vi "UI 3 Error.vi"(8 "error in (no error)":errorcluster, 11 "Data":variant) -> (0 "error out":errorcluster)   [LabVIEW 2018, in "Error Handler.lvlib"]
doc: "This subVI enqueues the named action in to the communications queue along with the input data."
uses:
  Error Handler.lvlib
  Private Controls/Module Data.ctl
  Private Controls/Module Action.ctl
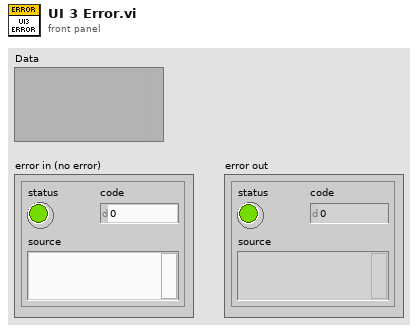
[diagram p1: front panel]
types:
  T1 = typedef "Error Handler.lvlib/Module Data.ctl" = cluster{"Data":variant, "Action":T2}
  T2 = typedef "Error Handler.lvlib/Module Action.ctl" = enum8{"Init", "Exit", "Controller Error", "UI1 Error", "UI2 Error", "UI3 Error", "File IO Error", "cRIO Error", "Calibration Error"}
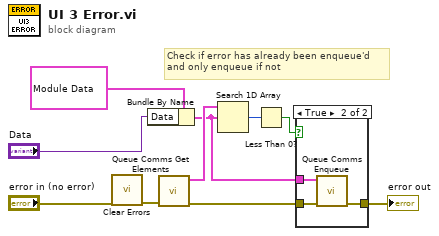
[diagram p0: block diagram]
diagram:
  # "Check if error has already been enqueue'd\nand only enqueue if not"
  n1 = call <vilib>:"Clear Errors.vi"("error in (no error)"="error in (no error)") -> ("error out"=w1:errorcluster)  [unwired: 5 in, 1 out]
  n2 = Bundle By Name(cluster=T1 {"Data"=variant, "Action"=enum."UI3 Error"} ("element"), "Data"="Data") -> (w5:T1)
  n3 = call "Queue Comms Get Elements.vi"("error in (no error)"=w1) -> ("error out"=w4:errorcluster, "elements"=w6:T1[])  [unwired: 9 in]
  n4 = Search 1D Array(1D array=w6, element=w5) -> (index of element=w7:i32)  [unwired: 1 in]
  n5 = Less Than 0?(x=w7) -> (x < 0?=w3:bool)
  n6 = case shown="True" w3 {
    tunnel: [w11 w14] -> w9
    tunnel: w5 -> [_ w13]
    tunnel: w4 -> [w11 w12]
    frame False {
    }
    frame True {
      n7 = call "Queue Comms Enqueue.vi"("error in (no error)"=w12, "element"=w13) -> ("error out"=w14:errorcluster)  [unwired: 9 in]
    }
  }
  "error out" <- w9
